vi "TDT-Init ActiveX.vi"(0 "TDT-Device Config":T1, 11 "error in (no error)":errorcluster) -> (4 "TDT-Device Config out":T1, 6 "RPcox":refnum<k7>, 8 "ZBUSx":refnum<k7>, 15 "error out":errorcluster)   [LabVIEW 2020]
uses:
  Typedefs/TDT-Device Config.ctl
  Typedefs/TDT-Output source.ctl
  Typedefs/TDT-Device ID.ctl
  Typedefs/TDT-Input source.ctl
  TDT-Globals.vi
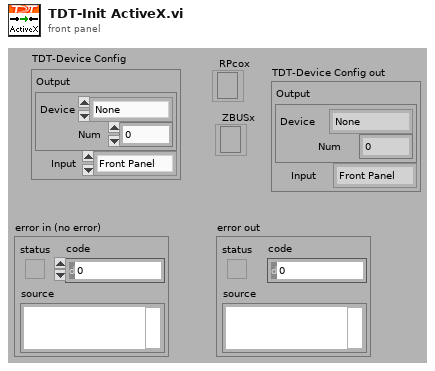
[diagram p1: front panel]
types:
  T1 = typedef "TDT-Device Config.ctl" = cluster{"Output":T2, "Input":T4}
  T2 = typedef "TDT-Output source.ctl" = cluster{"Device":T3, "Num":i32}
  T3 = typedef "TDT-Device ID.ctl" = enum16{"None", "PA5", "RP2", "RL2", "RA16", "RV8", "RX5", "RX6", "RX7", "RX8", "RZ2", "RZ5", "RZ6"}
  T4 = typedef "TDT-Input source.ctl" = enum16{"Front Panel", "RA4LI", "RA16LI"}
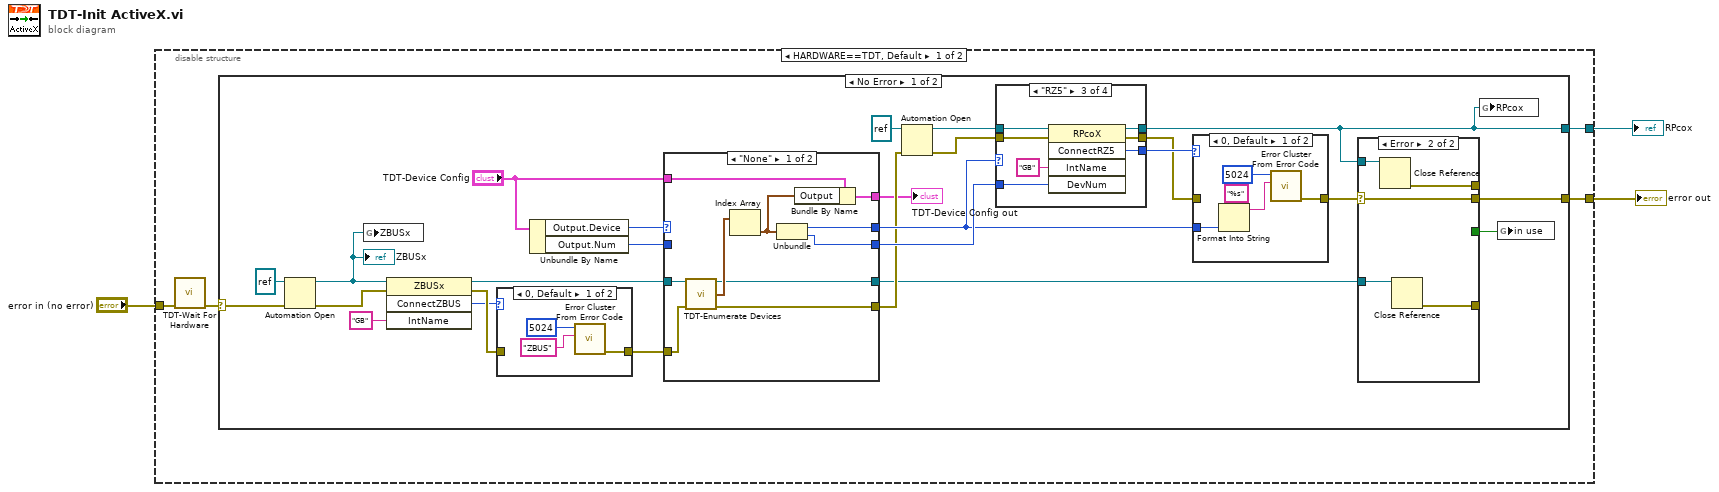
[diagram p0: block diagram]
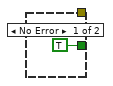
[diagram p2: hidden frame]
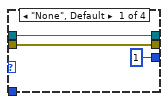
[diagram p5: hidden frame]
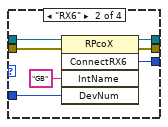
[diagram p6: hidden frame]
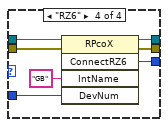
[diagram p7: hidden frame]
diagram:
  n1 = disable-structure shown="HARDWARE==TDT, Default" {
    disable-tunnel: [w6 _] -> w3
    disable-tunnel: "error in (no error)" -> [w5 w90]
    disable-tunnel: [w7 w90] -> w1
    frame condition #0 (active) {
      n2 = call "TDT-Wait For Hardware.vi"("error in (no error)"=w5) -> ("error out"=w4:errorcluster)  [unwired: 14 in]
      n3 = case shown="No Error" w4 {
        selector: w4 -> [w9 w89]
        tunnel: [w12 w89] -> w7
        tunnel: [w8 _] -> w6
        frame No Error {
          n4 = Automation Open(error in (no error)=w9, Automation Refnum=refnum<k7> refnum ("ZBUSXLib.ZBUSx")) -> (Automation Refnum=w20:refnum<k7>, error out=w23:errorcluster)  [unwired: 2 in]
          "ZBUSx" <- w20
          n5 = global write "TDT-Globals.vi" "ZBUSx"(w20) -> ()
          n6 = invoke class="ZBUSx" method="ConnectZBUS"(reference=w20, error in=w23, "IntName"="GB" ("ServerName")) -> (reference out=w22:refnum<k7>, error out=w32:errorcluster, "ConnectZBUS"=w31:i32)  [unwired: 1 in, 1 out]
          n7 = case shown="0, Default" w31 {
            tunnel: w32 -> [_ w58]
            tunnel: [w55 w58] -> w21
            frame 0, Default {
              n8 = call <vilib>:"Error Cluster From Error Code.vi"("error message (\"\")"="ZBUS" ("error message (\"\")"), "error code (0)"=5024) -> ("error out"=w55:errorcluster)  [unwired: 7 in]
            }
            frame 1 {
            }
          }
          n9 = Unbundle By Name("TDT-Device Config") -> ("Output.Device"=w25:T3, "Output.Num"=w24:i32)
          n10 = case shown="\"None\"" w25 {
            selector: w25 -> [_ w54]
            tunnel: w24 -> [_ w53]
            tunnel: w22 -> [w49 w50]
            tunnel: w21 -> [w48 w52]
            tunnel: [w45 w54] -> w18
            tunnel: [w44 w53] -> w19
            tunnel: [w47 w52] -> w17
            tunnel: "TDT-Device Config" -> [w43 w51]
            tunnel: [w41 w51] -> w15
            tunnel: [w40 w50] -> w11
            frame "None" {
              n11 = call "TDT-Enumerate Devices.vi"("ZBUSx In"=w49, "error in (no error)"=w48) -> ("ZBUSx Out"=w40:refnum<k7>, "Devices"=w46:T2[], "error out"=w47:errorcluster)  [unwired: 11 in]
              n12 = Index Array(array=w46) -> (element=w42:T2)  [unwired: 1 in]
              n13 = Unbundle(w42) -> ("Device"=w45:T3, "Num"=w44:i32)
              n14 = Bundle By Name(cluster=w43, "Output"=w42) -> (w41:T1)
            }
            frame "RX6", Default {
            }
          }
          "TDT-Device Config out" <- w15
          n15 = Automation Open(error in (no error)=w17, Automation Refnum=refnum<k7> refnum ("RPCOXLib.RPcoX")) -> (Automation Refnum=w29:refnum<k7>, error out=w28:errorcluster)  [unwired: 2 in]
          n16 = case shown="\"RZ5\"" w18 {
            tunnel: w29 -> [w60 w68 w75 w82]
            tunnel: w28 -> [w61 w66 w73 w80]
            tunnel: [1 ("ConnectRX6") w65 w72 w79] -> w27
            tunnel: [w61 w64 w71 w78] -> w26
            tunnel: [w60 w63 w70 w77] -> w8
            tunnel: w19 -> [_ w62 w69 w76]
            frame "None", Default {
            }
            frame "RX6" {
              n17 = invoke class="RPcoX" method="ConnectRX6"(reference=w68, error in=w66, "IntName"="GB", "DevNum"=w62) -> (reference out=w63:refnum<k7>, error out=w64:errorcluster, "ConnectRX6"=w65:i32)  [unwired: 1 in, 2 out]
            }
            frame "RZ5" {
              n18 = invoke class="RPcoX" method="ConnectRZ5"(reference=w75, error in=w73, "IntName"="GB", "DevNum"=w69) -> (reference out=w70:refnum<k7>, error out=w71:errorcluster, "ConnectRZ5"=w72:i32)  [unwired: 1 in, 2 out]
            }
            frame "RZ6" {
              n19 = invoke class="RPcoX" method="ConnectRZ6"(reference=w82, error in=w80, "IntName"="GB", "DevNum"=w76) -> (reference out=w77:refnum<k7>, error out=w78:errorcluster, "ConnectRZ6"=w79:i32)  [unwired: 1 in, 2 out]
            }
          }
          n20 = case shown="0, Default" w27 {
            tunnel: w26 -> [_ w88]
            tunnel: [w86 w88] -> w14
            tunnel: w18 -> [w85 _]
            frame 0, Default {
              n21 = Format Into String(format string="%s", w85) -> (resulting string=w84:string)  [unwired: 2 in, 1 out]
              n22 = call <vilib>:"Error Cluster From Error Code.vi"("error message (\"\")"=w84, "error code (0)"=5024) -> ("error out"=w86:errorcluster)  [unwired: 7 in]
            }
            frame 1 {
            }
          }
          n23 = case shown="Error" w14 {
            selector: w14 -> [_ w39]
            tunnel: [TRUE _] -> w13
            tunnel: [_ w39] -> w12
            tunnel: w8 -> [_ w38]
            tunnel: [_ w37] -> _
            tunnel: w11 -> [_ w36]
            tunnel: [_ w35] -> _
            frame No Error {
            }
            frame Error {
              n24 = Close Reference(reference=w38) -> (error out=w37:errorcluster)  [unwired: 1 in]
              n25 = Close Reference(reference=w36) -> (error out=w35:errorcluster)  [unwired: 1 in]
            }
          }
          n26 = global write "TDT-Globals.vi" "RPcox"(w8) -> ()
          n27 = global write "TDT-Globals.vi" "in use"(w13) -> ()
        }
        frame Error {
        }
      }
    }
    frame condition #1 {
    }
  }
  "error out" <- w1
  "RPcox" <- w3
